vi "ShowImage.vi"(2 "Color Table":T1(ring), 3 "Autoscale?":bool, 4 "Image":T2 {"Dialogs" format="%.0b"}) -> (0 "dimensions":cluster{"Witdh":i32, "Height":i32}, 1 "image":picture)   [LabVIEW 2024]
doc: "This VI is used to convert the Image Processing Toolkit “image” data type into the LabVIEW “image” data type used by indicators. This VI is essential to view images on the front panel."
uses:
  <userlib>/ImageProcessing/QTLIB_2595_LV86/QT_Image.ctl
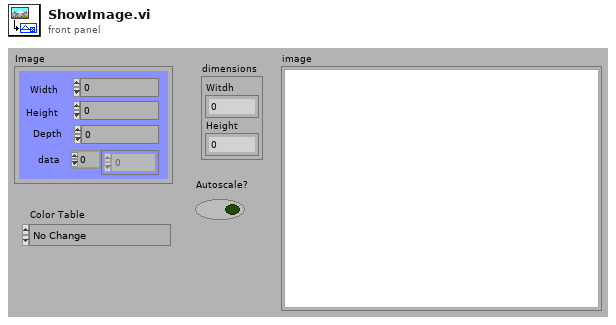
[diagram p1: front panel]
types:
  T1 = enum16{"No Change", "Apricot", "Carnation", "Ether", "Greyscale", "Greyscale-banded", "Hot Metal", "Lava Waves", "Mac", "Morning Glory", "Rainbow", "Rainbow-banded", "Rainbow-inverted", "Rainbow-striped", "Saturn", "Seismic", "Space"}
  T2 = typedef "QT_Image.ctl" = cluster{"Width":i32, "Height":i32, "Depth":i32, "data":u8[], "Compressed data":u8[], "Color table":u32[], "Duration":i32, "Options":i32, "Timestamp":i32, "ID":i32, "Reserved":i32, "Dialogs":u32}
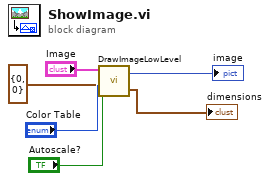
[diagram p0: block diagram]
diagram:
  n1 = call <userlib>:"DrawImageLowLevel.vi"("Image"="Image", "Position"=cluster{"left":i16, "top":i16} {"left"=0, "top"=0}, "Color Table"="Color Table", "Autoscale?"="Autoscale?") -> ("new picture"=→"image":picture, "dimensions"=→"dimensions":cluster{"Width":i32, "Height":i32})  [unwired: 1 in]
